vi "Create Controls.vi"(0 "VI in":refnum<vi>, 5 "Ctl Refnum":refnum<vi>, 7 "Control Label":string, 11 "error in (no error)":errorcluster) -> (15 "error out":errorcluster)   [LabVIEW 2021, in "Migrator.lvlib"]
uses:
  Migrator.lvlib
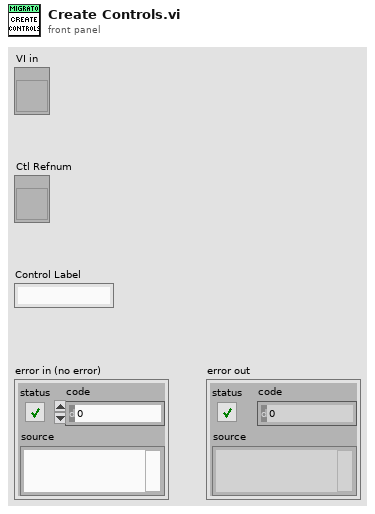
[diagram p1: front panel]
types:
  T1 = typedef "LVPositionTypeDef.ctl" = cluster{"Left":i32, "Top":i32}
  T2 = enum32{"not a typedef", "typedef", "strict typedef", "class private data"}
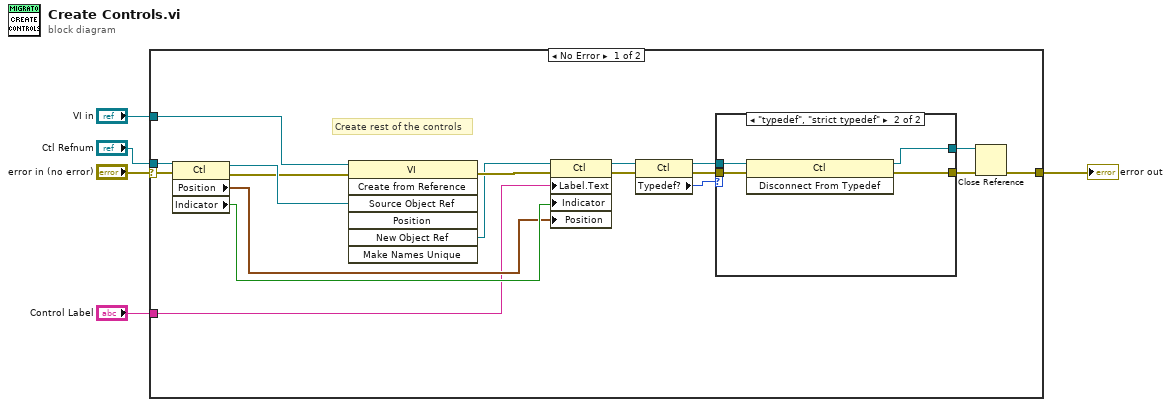
[diagram p0: block diagram]
diagram:
  n1 = case shown="No Error" "error in (no error)" {
    selector: "error in (no error)" -> [w19 w30]
    tunnel: "Ctl Refnum" -> [w18 _]
    tunnel: "Control Label" -> [w16 _]
    tunnel: [w14 w30] -> w2
    tunnel: "VI in" -> [w13 _]
    frame No Error {
      # "Create rest of the controls"
      n2 = property class="Ctl"(reference=w18, error in=w19) -> (reference out=w21:refnum<vi>, error out=w20:errorcluster, "Position"=w22:T1, "Indicator"=w23:bool)
      n3 = invoke class="VI" method="Create from Reference"(reference=w13, error in=w20, "Source Object Ref"=w21) -> (error out=w17:errorcluster, "New Object Ref"=w15:refnum<vi>)  [unwired: 4 in, 5 out]
      n4 = property class="Ctl"(reference=w15, error in=w17, "Label.Text"=w16, "Indicator"=w23, "Position"=w22) -> (reference out=w9:refnum<vi>, error out=w12:errorcluster)
      n5 = property class="Ctl"(reference=w9, error in=w12) -> (reference out=w8:refnum<vi>, error out=w10:errorcluster, "Typedef?"=w11:T2)
      n6 = case shown="\"typedef\", \"strict typedef\"" w11 {
        tunnel: w10 -> [w24 w29]
        tunnel: w8 -> [w25 w28]
        tunnel: [w24 w27] -> w7
        tunnel: [w25 w26] -> w6
        frame "not a typedef", Default {
        }
        frame "typedef", "strict typedef" {
          n7 = invoke class="Ctl" method="Disconnect From Typedef"(reference=w28, error in=w29) -> (reference out=w26:refnum<vi>, error out=w27:errorcluster)  [unwired: 1 in, 1 out]
        }
      }
      n8 = Close Reference(reference=w6, error in (no error)=w7) -> (error out=w14:errorcluster)
    }
    frame Error {
    }
  }
  "error out" <- w2
